vi "fluke_temp_reader.vi"(3 "error in (no error)":errorcluster, 4 "Bytes to Read":u32, 5 "COM Port In":refnum<visa-resource-name>) -> (0 "error out":errorcluster, 1 "Temp":dbl, 2 "COM Port Out":refnum<visa-resource-name>)   [LabVIEW 2010]
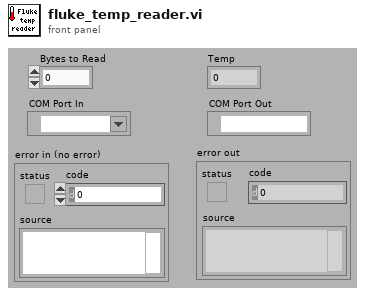
[diagram p1: front panel]
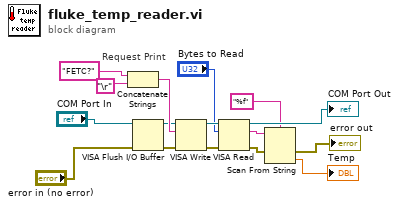
[diagram p0: block diagram]
diagram:
  # "Request Print"
  n1 = Concatenate Strings("FETC?", "\r") -> (w14:string)
  n2 = VISA Flush I/O Buffer(VISA resource name="COM Port In", error in (no error)="error in (no error)") -> (VISA resource name out=w11:refnum<visa-resource-name>, error out=w12:errorcluster)  [unwired: 1 in]
  n3 = VISA Write(VISA resource name=w11, write buffer=w14, error in (no error)=w12) -> (VISA resource name out=w15:refnum<visa-resource-name>, error out=w16:errorcluster)  [unwired: 1 out]
  n4 = VISA Read(VISA resource name=w15, byte count="Bytes to Read", error in (no error)=w16) -> (VISA resource name out=→"COM Port Out":refnum<visa-resource-name>, read buffer=w3:string, error out=w5:errorcluster)  [unwired: 1 out]
  n5 = Scan From String(format string="%f", input string=w3, error in=w5) -> (error out=→"error out":errorcluster, output 1=→"Temp":dbl)  [unwired: 2 in, 2 out]
